vi "Update Device.vi"(7 "Device in":refnum<class "Device.lvclass">, 8 "error in (no error)":errorcluster, 10 "Get Stack ID Response":T1) -> (0 "error out":errorcluster, 2 "Device out":refnum<class "Device.lvclass">)   [LabVIEW 2011, in "Tinkerforge.lvlib" / "Device.lvclass"]
doc: "This VI updates the device meta data received from the get stack ID request."
uses:
  Device.lvclass
  IP Connection/Type Definitions/Get Stack ID Response.ctl
  Type Definitions/Firmware Version.ctl
  Device.lvclass/Device.ctl
  IP Connection/IP Connection.lvclass
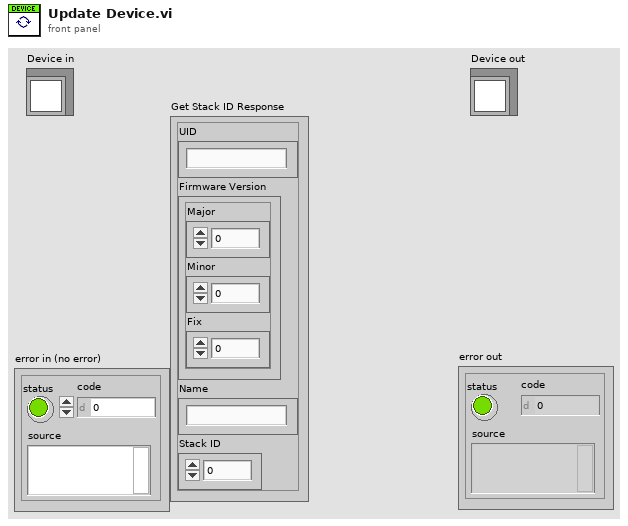
[diagram p1: front panel]
types:
  T1 = typedef "Tinkerforge.lvlib/IP Connection.lvclass/Get Stack ID Response.ctl" = cluster{"UID":string, "Firmware Version":T2, "Name":string, "Stack ID":u8}
  T2 = typedef "Tinkerforge.lvlib/Device.lvclass/Firmware Version.ctl" = cluster{"Major":u8, "Minor":u8, "Fix":u8}
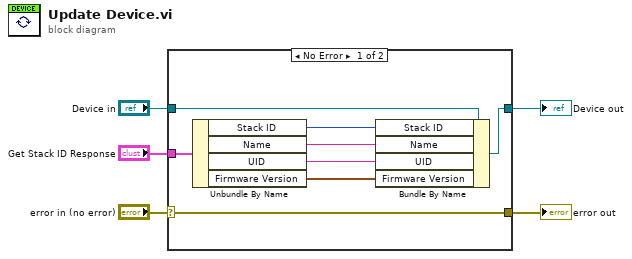
[diagram p0: block diagram]
diagram:
  n1 = case shown="No Error" "error in (no error)" {
    selector: "error in (no error)" -> [w13 w15]
    tunnel: [w13 w15] -> w4
    tunnel: [w11 w14] -> w2
    tunnel: "Device in" -> [w12 w14]
    tunnel: "Get Stack ID Response" -> [w10 _]
    frame No Error {
      n2 = Unbundle By Name(w10) -> ("Stack ID"=w9:u8, "Name"=w8:string, "UID"=w7:string, "Firmware Version"=w6:T2)
      n3 = Bundle By Name(cluster=w12, "Stack ID"=w9, "Name"=w8, "UID"=w7, "Firmware Version"=w6) -> (w11:refnum<class "Device.lvclass">)
    }
    frame Error {
    }
  }
  "error out" <- w4
  "Device out" <- w2
